vi "loadRepoCfgFile.vi"(8 "error in (no error)":errorcluster, 11 "path to XML document":path) -> (0 "error out":errorcluster, 3 "repoHandlers":refnum<class "repoHandler.lvclass">[](array[class]))   [LabVIEW 2013]
uses:
  repoHandler/repoHandler.lvclass
  hgHandler/hgHandler.lvclass
  svnHandler/svnHandler.lvclass
  <vilib>/xml/Load XML File.vi
  <vilib>/xml/NI_XML.lvlib
  <resource>/objmgr/DOMUserDefRef.rc
panel:
  out "parse errors":string
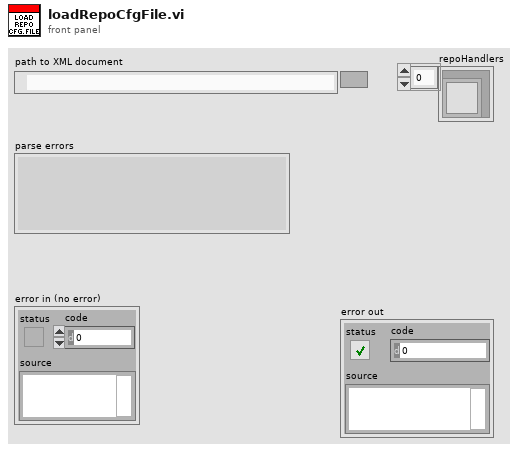
[diagram p1: front panel]
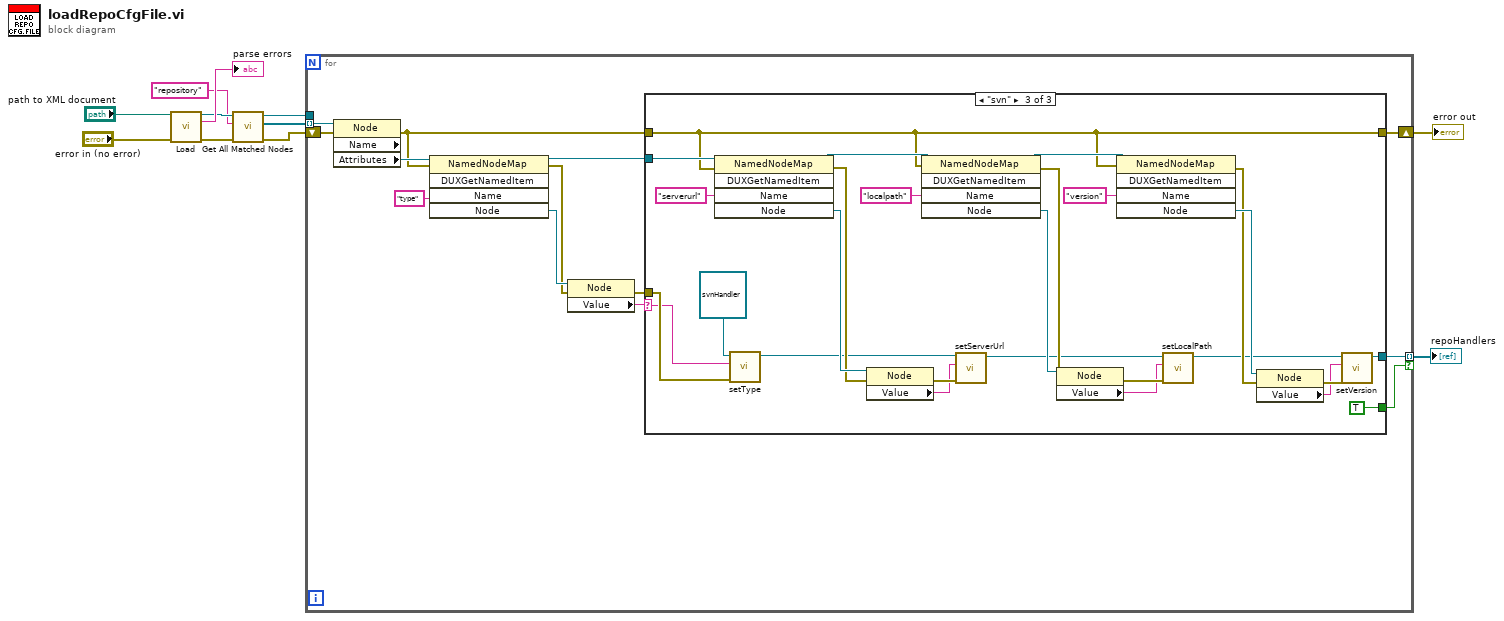
[diagram p0: block diagram]
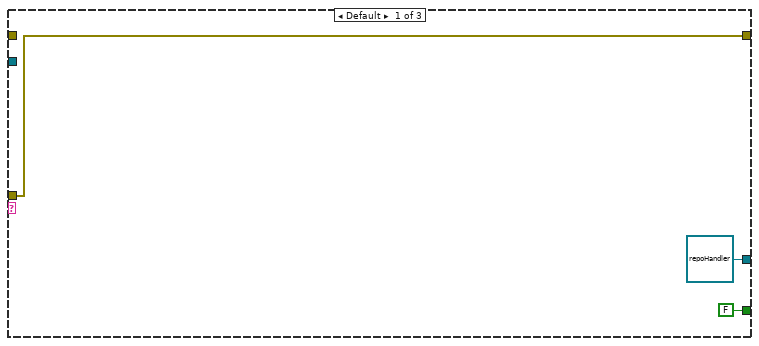
[diagram p2: hidden frame]
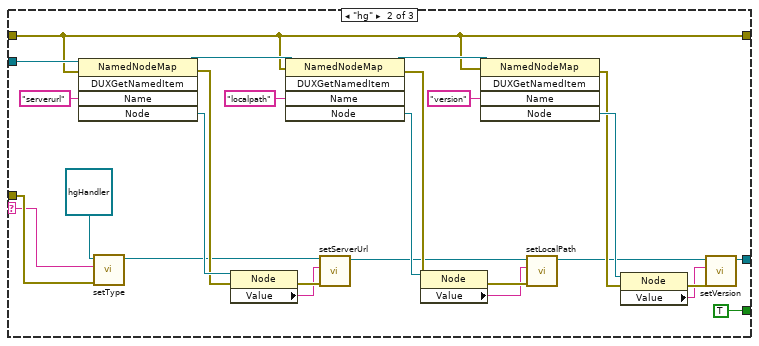
[diagram p3: hidden frame]
diagram:
  n1 = call-poly <vilib>:"Load.vi"("path to XML document"="path to XML document", "error in (no error)"="error in (no error)") -> ("DOM document out"=w9:refnum<k20>, "parse errors"=→"parse errors":string, "error out"=w6:errorcluster)  [unwired: 11 in]
  n2 = call <vilib>:"Get All Matched Nodes.vi"("error in (no error)"=w6, "XPath expression"="repository", "node in"=w9) -> ("error out"=w4:errorcluster, "node result array"=w7:refnum<k20>[], "node out"=w5:refnum<k20>)  [unwired: 6 in]
  n3 = for {
    tunnel: w7 -> [w24] mode=indexing
    tunnel: w5 -> [_]
    shift-right: [w15] -> w2
    shift-left: w4 -> [w19]
    tunnel: [w14] -> w1 mode=indexing if=w13
    n4 = property class="Node" props=["Name", "Attributes"](reference=w24, error in=w19) -> (error out=w17:errorcluster, "Attributes"=w23:refnum<k20>)  [unwired: 2 out]
    n5 = invoke class="NamedNodeMap" method="DUXGetNamedItem"(reference=w23, error in=w17, "Name"="type") -> (reference out=w20:refnum<k20>, error out=w18:errorcluster, "Node"=w21:refnum<k20>)  [unwired: 2 in, 2 out]
    n6 = property class="Node"(reference=w21, error in=w18) -> (error out=w12:errorcluster, "Value"=w16:string)  [unwired: 1 out]
    n7 = case shown="\"svn\"" w16 {
      selector: w16 -> [_ w30 w57]
      tunnel: w20 -> [_ w53 w80]
      tunnel: w17 -> [_ w36 w63]
      tunnel: [w25 w36 w63] -> w15
      tunnel: [refnum<class "repoHandler.lvclass"> refnum ("repoHandler out") w33 w60] -> w14
      tunnel: [FALSE TRUE TRUE] -> w13
      tunnel: w12 -> [w25 w31 w58]
      frame Default {
      }
      frame "hg" {
        n8 = invoke class="NamedNodeMap" method="DUXGetNamedItem"(reference=w53, error in=w36, "Name"="serverurl") -> (reference out=w51:refnum<k20>, error out=w45:errorcluster, "Node"=w48:refnum<k20>)  [unwired: 2 in, 2 out]
        n9 = call-dynamic "setType.vi"("error in (no error)"=w31, "Type"=w30, "repoHandler in"=refnum<class "hgHandler.lvclass"> refnum ("hgHandler.lvclass")) -> ("repoHandler out"=w29:refnum<class "hgHandler.lvclass">)  [unwired: 7 in, 1 out]
        n10 = property class="Node"(reference=w48, error in=w45) -> (error out=w42:errorcluster, "Value"=w41:string)  [unwired: 1 out]
        n11 = invoke class="NamedNodeMap" method="DUXGetNamedItem"(reference=w51, error in=w36, "Name"="localpath") -> (reference out=w49:refnum<k20>, error out=w44:errorcluster, "Node"=w47:refnum<k20>)  [unwired: 2 in, 2 out]
        n12 = call-dynamic "setServerUrl.vi"("error in (no error)"=w42, "serverUrl"=w41, "repoHandler in"=w29) -> ("repoHandler out"=w40:refnum<class "hgHandler.lvclass">)  [unwired: 7 in, 1 out]
        n13 = property class="Node"(reference=w47, error in=w44) -> (error out=w38:errorcluster, "Value"=w37:string)  [unwired: 1 out]
        n14 = invoke class="NamedNodeMap" method="DUXGetNamedItem"(reference=w49, error in=w36, "Name"="version") -> (error out=w43:errorcluster, "Node"=w46:refnum<k20>)  [unwired: 2 in, 3 out]
        n15 = call-dynamic "setLocalPath.vi"("error in (no error)"=w38, "localPath"=w37, "repoHandler in"=w40) -> ("repoHandler out"=w39:refnum<class "hgHandler.lvclass">)  [unwired: 7 in, 1 out]
        n16 = property class="Node"(reference=w46, error in=w43) -> (error out=w35:errorcluster, "Value"=w34:string)  [unwired: 1 out]
        n17 = call-dynamic "setVersion.vi"("error in (no error)"=w35, "setVersion"=w34, "repoHandler in"=w39) -> ("repoHandler out"=w33:refnum<class "hgHandler.lvclass">)  [unwired: 7 in, 1 out]
      }
      frame "svn" {
        n18 = invoke class="NamedNodeMap" method="DUXGetNamedItem"(reference=w80, error in=w63, "Name"="serverurl") -> (reference out=w78:refnum<k20>, error out=w72:errorcluster, "Node"=w75:refnum<k20>)  [unwired: 2 in, 2 out]
        n19 = call-dynamic "setType.vi"("error in (no error)"=w58, "Type"=w57, "repoHandler in"=refnum<class "svnHandler.lvclass"> refnum ("svnHandler.lvclass")) -> ("repoHandler out"=w56:refnum<class "svnHandler.lvclass">)  [unwired: 7 in, 1 out]
        n20 = property class="Node"(reference=w75, error in=w72) -> (error out=w69:errorcluster, "Value"=w68:string)  [unwired: 1 out]
        n21 = invoke class="NamedNodeMap" method="DUXGetNamedItem"(reference=w78, error in=w63, "Name"="localpath") -> (reference out=w76:refnum<k20>, error out=w71:errorcluster, "Node"=w74:refnum<k20>)  [unwired: 2 in, 2 out]
        n22 = call-dynamic "setServerUrl.vi"("error in (no error)"=w69, "serverUrl"=w68, "repoHandler in"=w56) -> ("repoHandler out"=w67:refnum<class "svnHandler.lvclass">)  [unwired: 7 in, 1 out]
        n23 = property class="Node"(reference=w74, error in=w71) -> (error out=w65:errorcluster, "Value"=w64:string)  [unwired: 1 out]
        n24 = invoke class="NamedNodeMap" method="DUXGetNamedItem"(reference=w76, error in=w63, "Name"="version") -> (error out=w70:errorcluster, "Node"=w73:refnum<k20>)  [unwired: 2 in, 3 out]
        n25 = call-dynamic "setLocalPath.vi"("error in (no error)"=w65, "localPath"=w64, "repoHandler in"=w67) -> ("repoHandler out"=w66:refnum<class "svnHandler.lvclass">)  [unwired: 7 in, 1 out]
        n26 = property class="Node"(reference=w73, error in=w70) -> (error out=w62:errorcluster, "Value"=w61:string)  [unwired: 1 out]
        n27 = call-dynamic "setVersion.vi"("error in (no error)"=w62, "setVersion"=w61, "repoHandler in"=w66) -> ("repoHandler out"=w60:refnum<class "svnHandler.lvclass">)  [unwired: 7 in, 1 out]
      }
    }
  }
  "error out" <- w2
  "repoHandlers" <- w1
